vi "z alloc layout loan.vi"(8 "error in (no error)":errorcluster, 11 "this_":cluster{}) -> (0 "error out":errorcluster, 3 "function return":u32)   [LabVIEW 2021, in "zenohc.lvlib"]
doc: "ZENOHC_API const z_loaned_alloc_layout_t *z_alloc_layout_loan(const z_owned_alloc_layout_t *this_);"
uses:
  zenohc.lvlib
  zenohc.dll
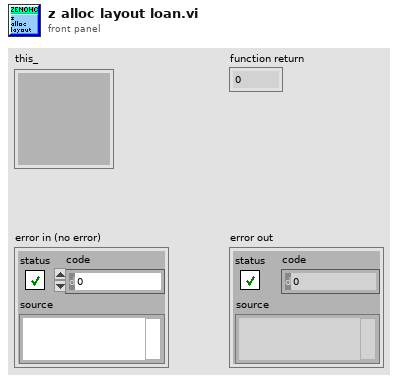
[diagram p1: front panel]
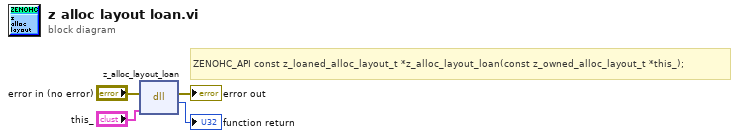
[diagram p0: block diagram]
diagram:
  # "ZENOHC_API const z_loaned_alloc_layout_t *z_alloc_layout_loan(const z_owned_alloc_layout_t *this_);"
  n1 = dll-call lib="D:/dev/zenoh_labview/zenohc/zenohc.*" fn="z_alloc_layout_loan"(error in="error in (no error)", "this_"="this_") -> (error out=→"error out":errorcluster, →"function return":u32)  [unwired: 3 in, 1 out]
